vi "macro_DigSeqLogic_OneShot.vi"   [LabVIEW 2019, in "Trajectory_Library.lvlib"]
uses:
  Trajectory_Library.lvlib
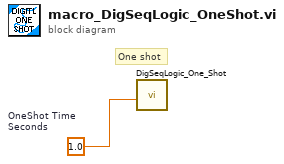
[diagram p0: block diagram]
diagram:
  w1 = 1.0  # OneShot Time Seconds
  # "One shot"
  n1 = call "DigSeqLogic_One_Shot.vi"("OneShot"=w1) -> ()  [unwired: 9 in, 2 out]
